vi "AllSensors.vi"(6 "sensor":u16, 8 "String in":string, 9 "Port 2":string, 10 "note (input a number)":string, 11 "Port":string) -> (3 "String out":string)   [LabVIEW 2022 SP3]
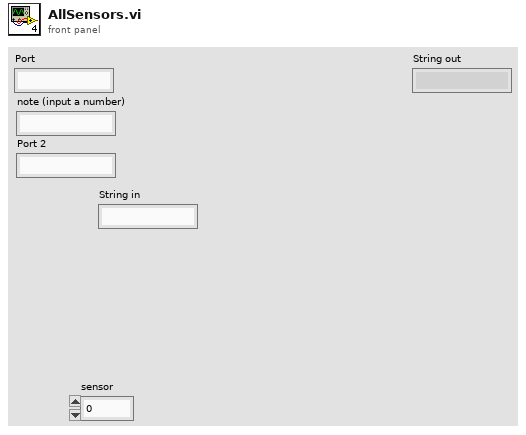
[diagram p1: front panel]
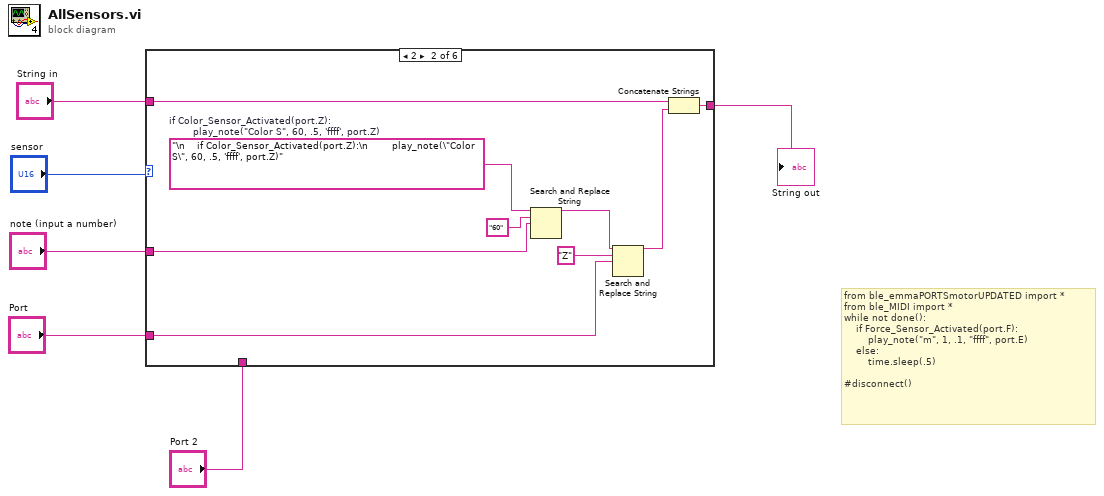
[diagram p0: block diagram]
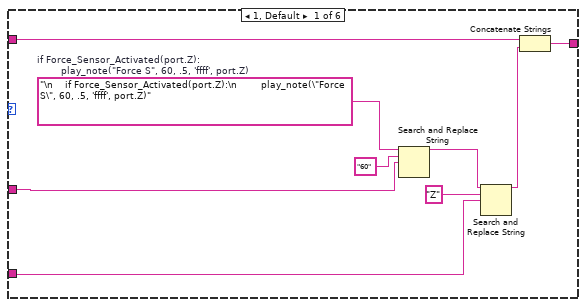
[diagram p2: hidden frame]
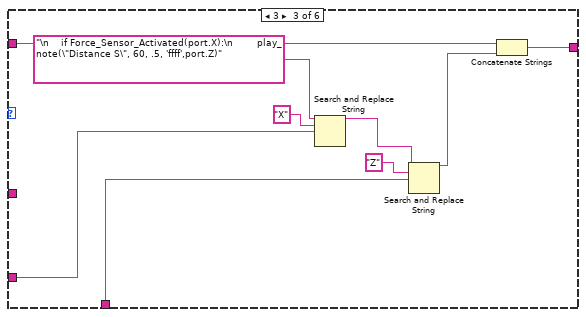
[diagram p3: hidden frame]
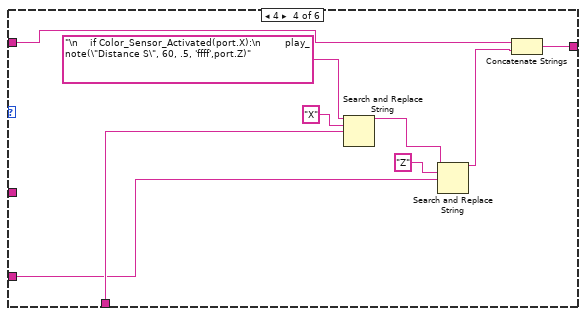
[diagram p4: hidden frame]
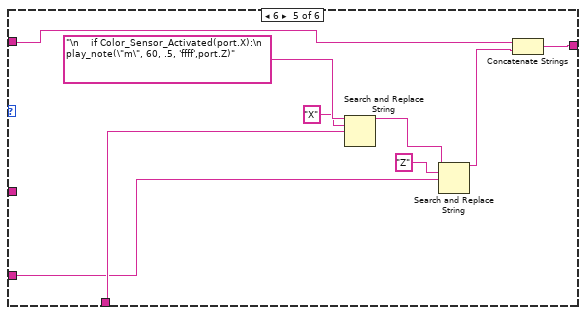
[diagram p5: hidden frame]
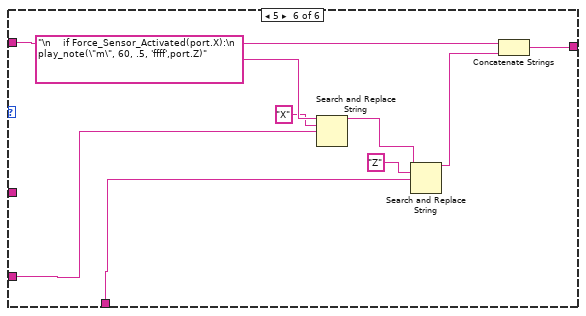
[diagram p6: hidden frame]
diagram:
  # "from ble_emmaPORTSmotorUPDATED import *\nfrom ble_MIDI import *\nwhile not done():\n    if Force_Sensor_Activated(port.F):\n        play_note(\"m\", 1, .1, \"ffff\", port.E)\n    else:\n        time.sleep(.5)\n   \n#disconnect()"
  n1 = case shown="2" "sensor" {
    tunnel: "String in" -> [w8 w24 w25 w34 w46 w53]
    tunnel: "note (input a number)" -> [w9 w21 _ _ _ _]
    tunnel: "Port" -> [w10 w20 w32 w37 w43 w54]
    tunnel: [w7 w16 w27 w36 w45 w52] -> w6
    tunnel: "Port 2" -> [_ _ w30 w38 w44 w55]
    frame 1, Default {
      w15 = "\n    if Force_Sensor_Activated(port.Z):\n        play_note(\"Force S\", 60, .5, 'ffff', port.Z)"  # if Force_Sensor_Activated(port.Z):         play_note("Force S", 60, .5, 'ffff', port.Z)
      n2 = Search and Replace String(input string=w15, search string="60", replace string=w9) -> (result string=w14:string)  [unwired: 5 in, 3 out]
      n3 = Search and Replace String(input string=w14, search string="Z", replace string=w10) -> (result string=w11:string)  [unwired: 5 in, 3 out]
      n4 = Concatenate Strings(w8, w11) -> (w7:string)
    }
    frame 2 {
      w23 = "\n    if Color_Sensor_Activated(port.Z):\n        play_note(\"Color S\", 60, .5, 'ffff', port.Z)"  # if Color_Sensor_Activated(port.Z):         play_note("Color S", 60, .5, 'ffff', port.Z)
      n5 = Search and Replace String(input string=w23, search string="60", replace string=w21) -> (result string=w22:string)  [unwired: 5 in, 3 out]
      n6 = Search and Replace String(input string=w22, search string="Z", replace string=w20) -> (result string=w17:string)  [unwired: 5 in, 3 out]
      n7 = Concatenate Strings(w24, w17) -> (w16:string)
    }
    frame 3 {
      n8 = Search and Replace String(input string="\n    if Force_Sensor_Activated(port.X):\n        play_note(\"Distance S\", 60, .5, 'ffff',port.Z)", search string="X", replace string=w32) -> (result string=w31:string)  [unwired: 5 in, 3 out]
      n9 = Search and Replace String(input string=w31, search string="Z", replace string=w30) -> (result string=w26:string)  [unwired: 5 in, 3 out]
      n10 = Concatenate Strings(w25, w26) -> (w27:string)
    }
    frame 4 {
      n11 = Search and Replace String(input string="\n    if Color_Sensor_Activated(port.X):\n        play_note(\"Distance S\", 60, .5, 'ffff',port.Z)", search string="X", replace string=w38) -> (result string=w41:string)  [unwired: 5 in, 3 out]
      n12 = Search and Replace String(input string=w41, search string="Z", replace string=w37) -> (result string=w35:string)  [unwired: 5 in, 3 out]
      n13 = Concatenate Strings(w34, w35) -> (w36:string)
    }
    frame 6 {
      n14 = Search and Replace String(input string="\n    if Color_Sensor_Activated(port.X):\n        play_note(\"m\", 60, .5, 'ffff',port.Z)", search string="X", replace string=w44) -> (result string=w50:string)  [unwired: 5 in, 3 out]
      n15 = Search and Replace String(input string=w50, search string="Z", replace string=w43) -> (result string=w51:string)  [unwired: 5 in, 3 out]
      n16 = Concatenate Strings(w46, w51) -> (w45:string)
    }
    frame 5 {
      n17 = Search and Replace String(input string="\n    if Force_Sensor_Activated(port.X):\n        play_note(\"m\", 60, .5, 'ffff',port.Z)", search string="X", replace string=w54) -> (result string=w59:string)  [unwired: 5 in, 3 out]
      n18 = Search and Replace String(input string=w59, search string="Z", replace string=w55) -> (result string=w60:string)  [unwired: 5 in, 3 out]
      n19 = Concatenate Strings(w53, w60) -> (w52:string)
    }
  }
  "String out" <- w6
